vi "Final Project.vi"() -> ()   [LabVIEW 2017]
panel:
  out "?":cluster{"Answer Indicator":u32}
  in  "Input your Initial Guess\n(Between 1-10)":dbl=1.0 min=1.0 max=10.0 step=1.0 format="%#_3g"
  # "Jay Patel\nDr. Kaputa\nBME 3120\n26 April 2018\n\nThis VI lets the user play a guessing game. \nThe user can input a number between 1-10.\nThe VI will say if it is too high, too low, or correct.\nDepending on the result, the LED will change color: red, yellow, or green, respectively.\nThe user can either play again or end it.\nThe VI will ask the user to save the results. The Final Project Read VI can read the results."
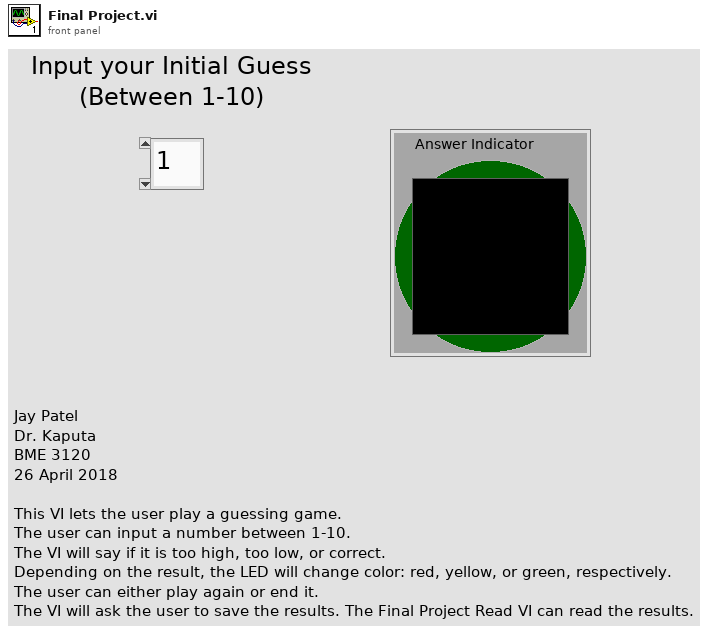
[diagram p1: front panel]
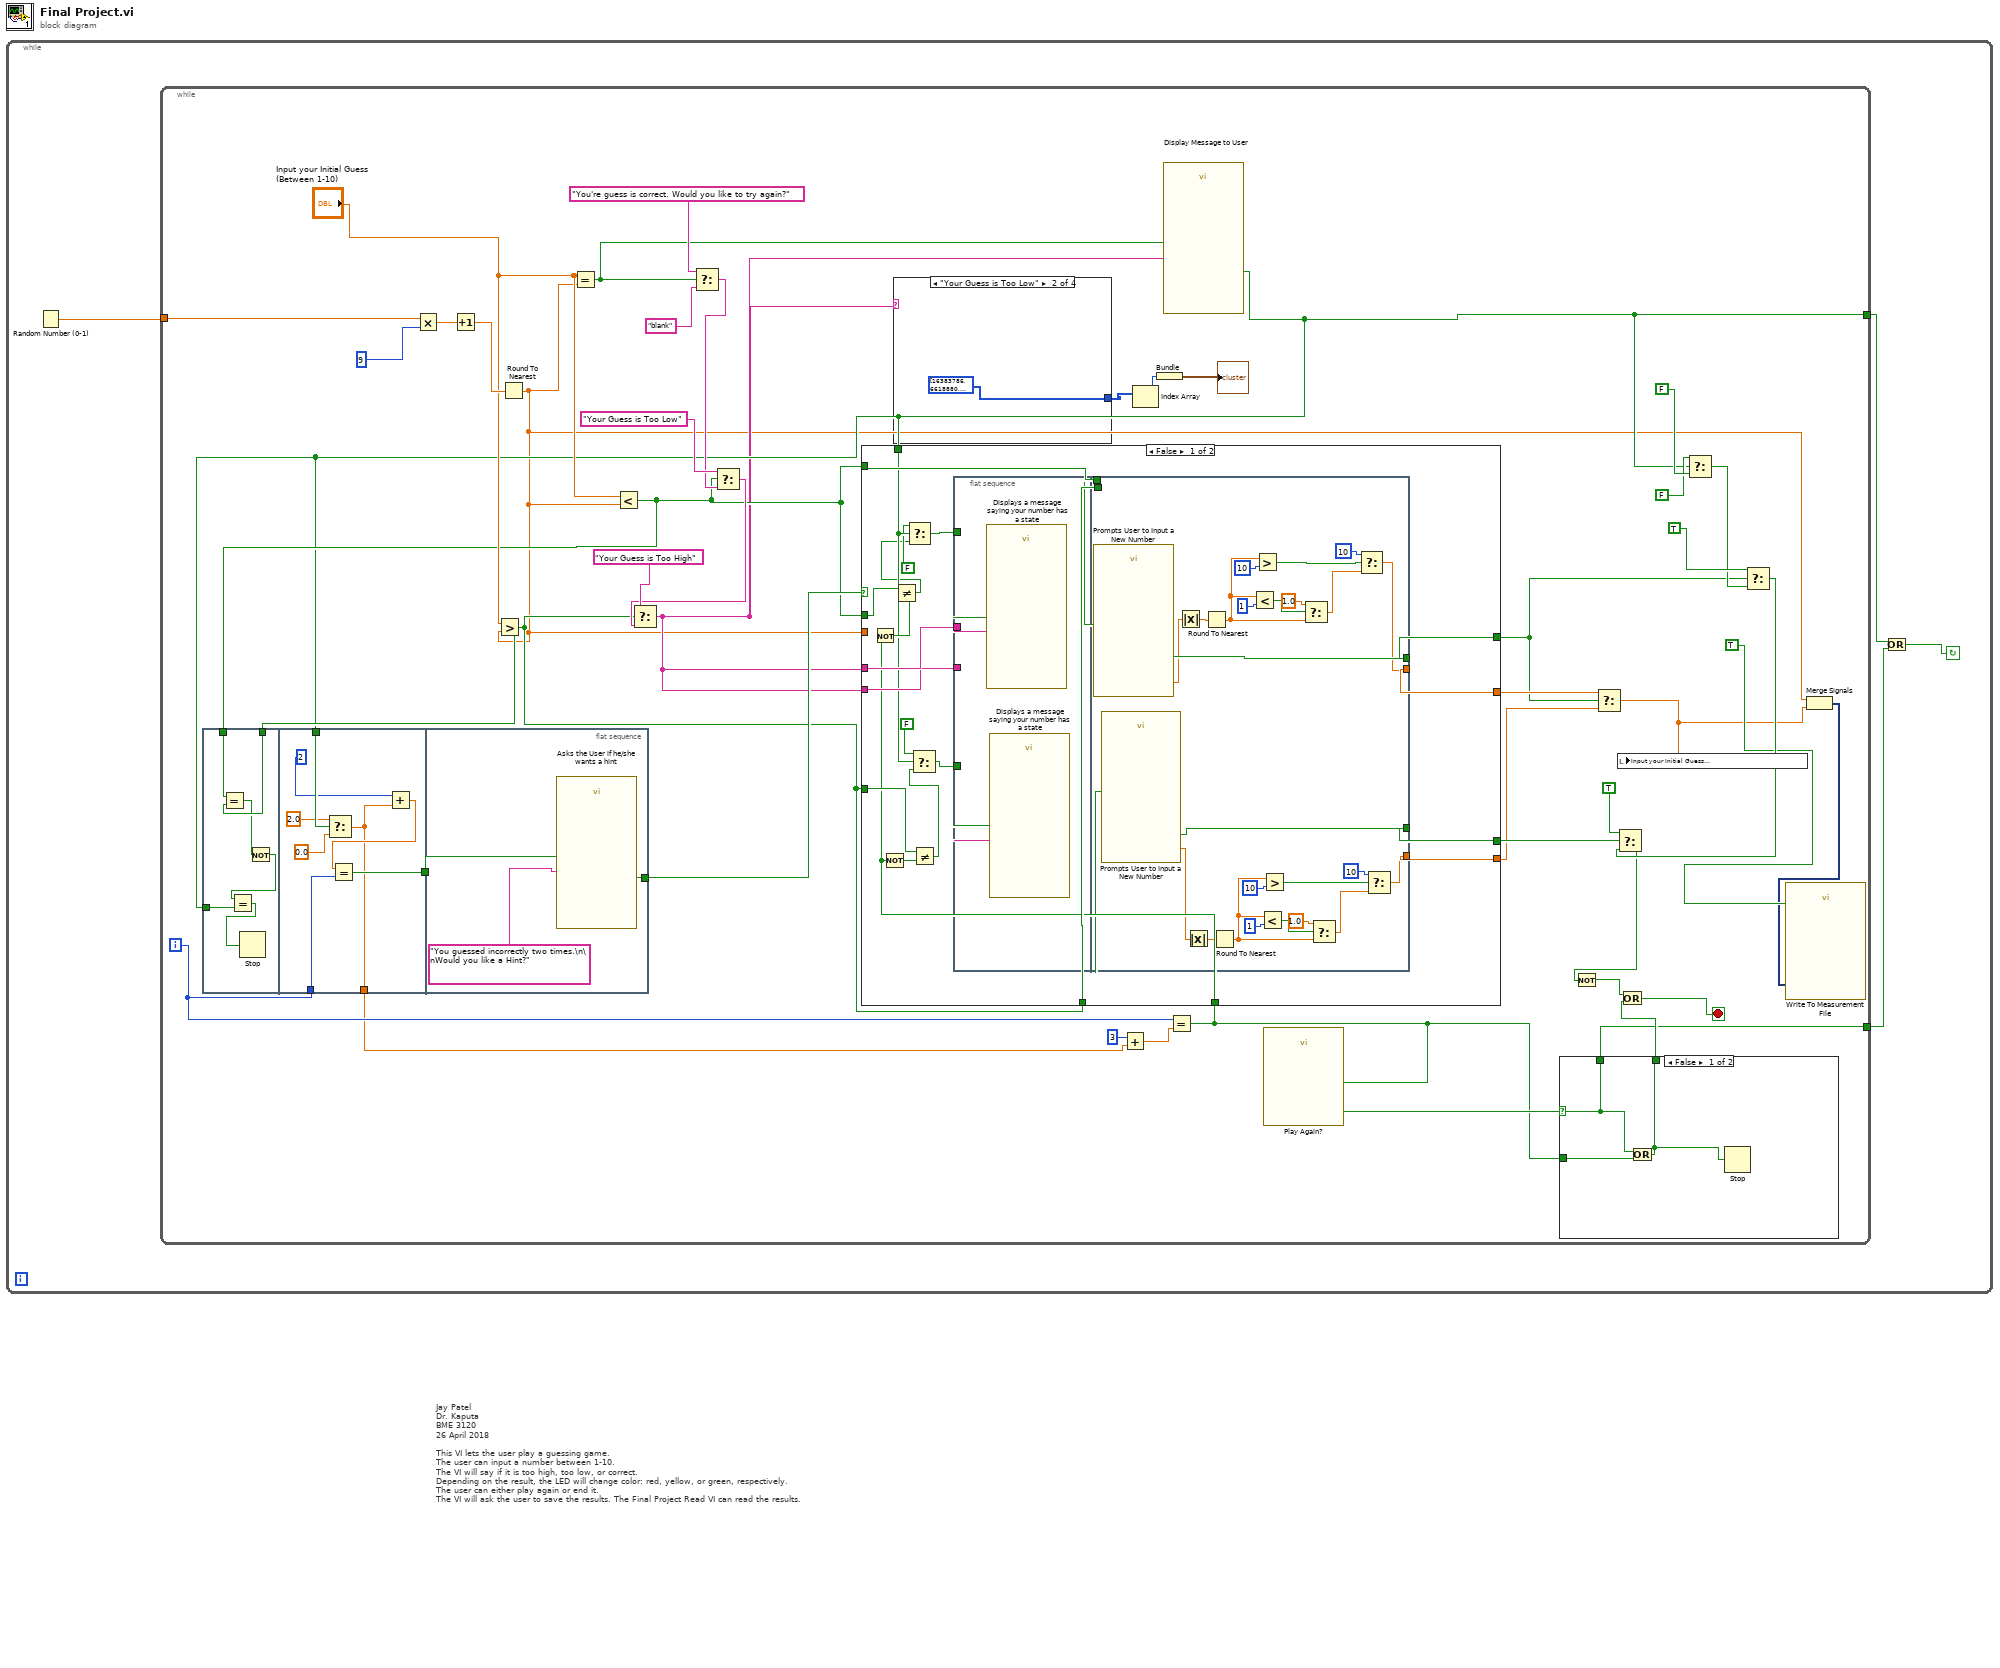
[diagram p0: block diagram]
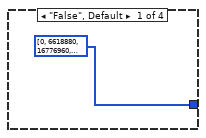
[diagram p2: hidden frame]
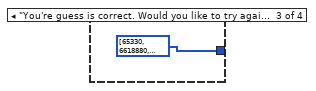
[diagram p3: hidden frame]
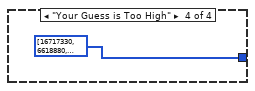
[diagram p4: hidden frame]
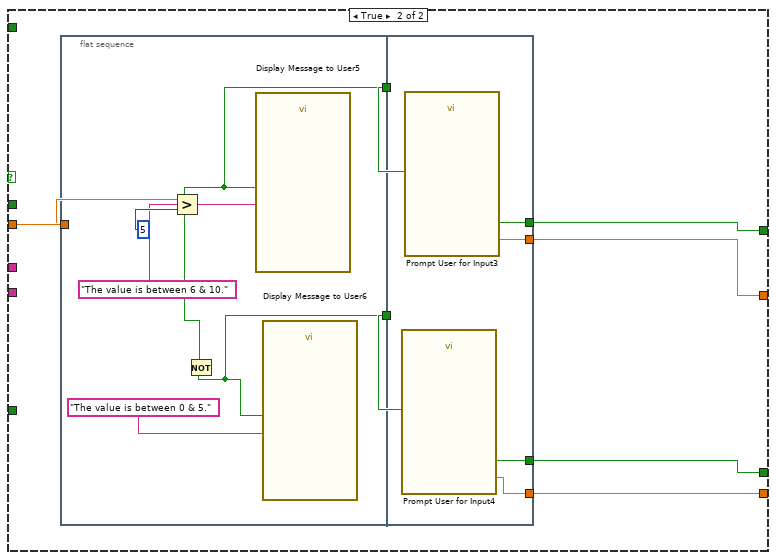
[diagram p6: hidden frame]
diagram:
  # "Jay Patel\nDr. Kaputa\nBME 3120\n26 April 2018\n\nThis VI lets the user play a guessing game. \nThe user can input a number between 1-10.\nThe VI will say if it is too high, too low, or correct.\nDepending on the result, the LED will change color: red, yellow, or green, respectively.\nThe user can either play again or end it.\nThe VI will ask the user to save the results. The Final Project Read VI can read the results."
  n1 = while {
    stop <- w3 continue-if-true
    n2 = Random Number (0-1)() -> (number: 0 to 1=w1:dbl)
    n3 = while {
      tunnel: w1 -> [w9]
      tunnel: [w14] -> w4
      tunnel: [w18] -> w2
      i -> [w28]
      stop <- w32 stop-if-true
      n4 = flat-sequence {
        tunnel: w16 -> [w64]
        tunnel: w15 -> [w63]
        tunnel: w14 -> [w60]
        tunnel: w14 -> [w70]
        tunnel: w28 -> [w67]
        tunnel: [w66] -> w27
        tunnel: [w65] -> w25
        tunnel: w27 -> [w75]
        tunnel: [w74] -> w19
        frame #0 {
          n5 = Equal?(x=w64, y=w63) -> (x = y?=w62:bool)
          n6 = Not(x=w62) -> (.not. x?=w61:bool)
          n7 = Equal?(x=w61, y=w60) -> (x = y?=w59:bool)
          n8 = Stop(stop? (T)=w59) -> ()
        }
        frame #1 {
          n9 = Select(t=2.0, s=w70, f=0.0) -> (s? t:f=w65:dbl)
          n10 = Add(x=2, y=w65) -> (x+y=w72:dbl)
          n11 = Equal?(x=w72, y=w67) -> (x = y?=w66:bool)
        }
        frame #2 {
          n12 = call "Asks the User if he/she wants a hint"("Enable"=w75, "Message"="You guessed incorrectly two times.\n\nWould you like a Hint?") -> ("Yes"=w74:bool)  [unwired: 8 in, 1 out]
        }
      }
      n13 = Multiply(x=w9, y=9) -> (x*y=w49:dbl)
      n14 = Increment(x=w49) -> (x+1=w48:dbl)
      n15 = Round To Nearest(number=w48) -> (nearest integer value=w6:dbl)
      n16 = Greater?(x="Input your Initial Guess\n(Between 1-10)", y=w6) -> (0:w15:bool)
      n17 = Equal?(x="Input your Initial Guess\n(Between 1-10)", y=w6) -> (x = y?=w36:bool)
      n18 = Less?(x="Input your Initial Guess\n(Between 1-10)", y=w6) -> (x < y?=w16:bool)
      n19 = Select(t="You're guess is correct. Would you like to try again?", s=w36, f="blank") -> (s? t:f=w43:string)
      n20 = Select(t="Your Guess is Too Low", s=w16, f=w43) -> (s? t:f=w42:string)
      n21 = Select(t="Your Guess is Too High", s=w15, f=w42) -> (s? t:f=w13:string)
      n22 = case shown="\"Your Guess is Too Low\"" w13 {
        tunnel: [u32[] [0, 6618880, 16776960, 16711680] u32[] [16383786, 6618880, 16776960, 16711680] u32[] [65330, 6618880, 16776960, 16711680] u32[] [16717330, 6618880, 16776960, 16711680]] -> w11
        frame "False", Default {
        }
        frame "Your Guess is Too Low" {
        }
        frame "You're guess is correct. Would you like to try again?" {
        }
        frame "Your Guess is Too High" {
        }
      }
      n23 = Add(x=3 ("y"), y=w25) -> (x+y=w24:dbl)
      n24 = Index Array(array=w11) -> (element=w10:u32)  [unwired: 1 in]
      n25 = Bundle(w10) -> (→"?":cluster{u32})  [unwired: 1 in]
      n26 = call "Display Message to User"("Enable"=w36, "Message"=w13) -> ("Yes"=w14:bool)  [unwired: 8 in, 1 out]
      n27 = Equal?(x=w28, y=w24) -> (x = y?=w17:bool)
      n28 = case shown="False" w19 {
        tunnel: w6 -> [_ w132]
        tunnel: w16 -> [w84 _]
        tunnel: w13 -> [w95 _]
        tunnel: w15 -> [w86 _]
        tunnel: w13 -> [w94 _]
        tunnel: w16 -> [w93 _]
        tunnel: w15 -> [w92 _]
        tunnel: [w91 w129] -> w31
        tunnel: [w90 w130] -> w29
        tunnel: [w89 w127] -> w30
        tunnel: [w88 w126] -> w35
        tunnel: w17 -> [w85 _]
        tunnel: w14 -> [w81 _]
        frame False {
          n29 = Not(x=w85) -> (.not. x?=w83:bool)
          n30 = Not(x=w85) -> (.not. x?=w87:bool)
          n31 = Not Equal?(x=w84, y=w83) -> (x != y?=w78:bool)
          n32 = Select(t=FALSE ("f"), s=w81, f=w78) -> (s? t:f=w82:bool)
          n33 = Not Equal?(x=w86, y=w87) -> (x != y?=w76:bool)
          n34 = Select(t=FALSE ("f"), s=w81, f=w76) -> (s? t:f=w80:bool)
          n35 = flat-sequence {
            tunnel: w95 -> [w99]
            tunnel: w80 -> [w96]
            tunnel: w94 -> [w98]
            tunnel: w82 -> [w97]
            tunnel: w93 -> [w125]
            tunnel: [w116] -> w91
            tunnel: [w124] -> w90
            tunnel: w92 -> [w123]
            tunnel: [w112] -> w89
            tunnel: [w122] -> w88
            frame #0 {
              n36 = call "Displays a message saying your number has a state"("Enable"=w97, "Message"=w99) -> ()  [unwired: 8 in, 2 out]
              n37 = call "Displays a message saying your number has a state"("Enable"=w96, "Message"=w98) -> ()  [unwired: 8 in, 2 out]
            }
            frame #1 {
              n38 = call "Prompts User to Input a New Number"("Enable"=w125) -> ("Input a New Number between 1 & 10"=w121:dbl, "OK"=w124:bool)  [unwired: 16 in, 1 out]
              n39 = call "Prompts User to Input a New Number"("Enable"=w123) -> ("Input a New Number between 1 & 10"=w111:dbl, "OK"=w122:bool)  [unwired: 16 in, 1 out]
              n40 = Absolute Value(x=w121) -> (abs(x)=w120:dbl)
              n41 = Absolute Value(x=w111) -> (abs(x)=w109:dbl)
              n42 = Round To Nearest(number=w120) -> (nearest integer value=w101:dbl)
              n43 = Round To Nearest(number=w109) -> (nearest integer value=w106:dbl)
              n44 = Less?(x=w101, y=1) -> (x < y?=w103:bool)
              n45 = Greater?(x=w101, y=10) -> (0:w118:bool)
              n46 = Less?(x=w106, y=1) -> (x < y?=w108:bool)
              n47 = Greater?(x=w106, y=10) -> (0:w114:bool)
              n48 = Select(t=1.0, s=w103, f=w101) -> (s? t:f=w100:dbl)
              n49 = Select(t=1.0, s=w108, f=w106) -> (s? t:f=w105:dbl)
              n50 = Select(t=10, s=w118, f=w100) -> (s? t:f=w116:dbl)
              n51 = Select(t=10, s=w114, f=w105) -> (s? t:f=w112:dbl)
            }
          }
        }
        frame True {
          n52 = flat-sequence {
            tunnel: w132 -> [w138]
            tunnel: [w134] -> w131
            tunnel: [w133] -> w128
            tunnel: w131 -> [w144]
            tunnel: [w143] -> w130
            tunnel: [w142] -> w129
            tunnel: w128 -> [w141]
            tunnel: [w140] -> w127
            tunnel: [w139] -> w126
            frame #0 {
              n53 = Greater?(x=w138, y=5) -> (0:w134:bool)
              n54 = Not(x=w134) -> (.not. x?=w133:bool)
              n55 = call "Display Message to User5"("Enable"=w134, "Message"="The value is between 6 & 10.") -> ()  [unwired: 8 in, 2 out]
              n56 = call "Display Message to User6"("Enable"=w133, "Message"="The value is between 0 & 5.") -> ()  [unwired: 8 in, 2 out]
            }
            frame #1 {
              n57 = call "Prompt User for Input4"("Enable"=w141) -> ("Input a New Number"=w140:dbl, "OK"=w139:bool)  [unwired: 16 in, 1 out]
              n58 = call "Prompt User for Input3"("Enable"=w144) -> ("Input a New Number"=w142:dbl, "OK"=w143:bool)  [unwired: 16 in, 1 out]
            }
          }
        }
      }
      n59 = call "Play Again?"("Enable"=w17) -> ("Yes"=w21:bool)  [unwired: 9 in, 1 out]
      n60 = case shown="False" w21 {
        selector: w21 -> [w56 w58]
        tunnel: [w55 w58] -> w20
        tunnel: [w56 w58] -> w18
        tunnel: w17 -> [w57 _]
        frame False {
          n61 = Or(x=w56, y=w57) -> (x .or. y?=w55:bool)
          n62 = Stop(stop? (T)=w55) -> ()
        }
        frame True {
        }
      }
      n63 = Select(t=w31, s=w29, f=w30) -> (s? t:f=w5:dbl)
      n64 = local write "Input your Initial Guess\n(Between 1-10)"(w5) -> ()
      n65 = Select(t=FALSE, s=w14, f=FALSE) -> (s? t:f=w38:bool)
      n66 = Select(t=TRUE, s=w29, f=w38) -> (s? t:f=w37:bool)
      n67 = Select(t=TRUE, s=w35, f=w37) -> (s? t:f=w34:bool)
      n68 = Not(x=w34) -> (.not. x?=w33:bool)
      n69 = Or(x=w33, y=w20) -> (x .or. y?=w32:bool)
      n70 = Merge Signals(w6, w5) -> (w7:dynamicdata)
      n71 = call "Write To Measurement File"("Signals"=w7, "Enable"=TRUE) -> ()  [unwired: 15 in, 3 out]
    }
    n72 = Or(x=w4, y=w2) -> (x .or. y?=w3:bool)
  }
